vi "Msg.vi"(7 "jettl in":refnum<class "jettl.lvclass">, 11 "Template Msg Strategy in":refnum<class "Template Msg Strategy.lvclass">) -> (5 "jettl out":refnum<class "jettl.lvclass">)   [LabVIEW 2021, in "jettl Msg Template.lvlib" / "Template Msg Strategy.lvclass"]
uses:
  Template Msg Strategy.lvclass
  <vilib>/Nathan Davis/jettl/jettl/jettl/jettl.lvclass
  jettl Msg Template/jettl Msg Template.lvclass
  Template Msg Strategy.lvclass/Template Msg Strategy.ctl
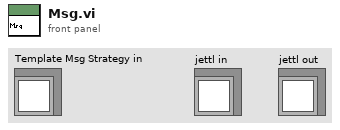
[diagram p1: front panel]
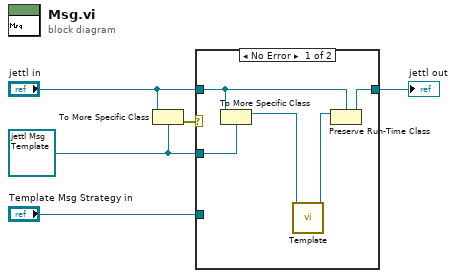
[diagram p0: block diagram]
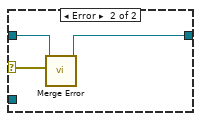
[diagram p2: hidden frame]
diagram:
  w2 = refnum<class "jettl Msg Template.lvclass"> refnum ("jettl Msg Template")
  n1 = To More Specific Class(target class=w2, reference="jettl in") -> (error out=w5:errorcluster)  [unwired: 1 in, 1 out]
  n2 = case shown="No Error" w5 {
    selector: w5 -> [_ w12]
    tunnel: [w8 w11] -> w3
    tunnel: "jettl in" -> [w9 w13]
    tunnel: w2 -> [w10 _]
    tunnel: "Template Msg Strategy in" -> [_ _]
    frame No Error {
      n3 = To More Specific Class(target class=w10, reference=w9) -> (specific class reference=w7:refnum<class "jettl Msg Template.lvclass">)  [unwired: 1 in, 1 out]
      n4 = call-dynamic "Template.vi"("jettl Msg Template in"=w7) -> ("jettl Msg Template out"=w6:refnum<class "jettl Msg Template.lvclass">)  [unwired: 10 in]
      n5 = Preserve Run-Time Class(object in=w6, 2:w9) -> (object out=w8:refnum<class "jettl.lvclass">)  [unwired: 1 in, 1 out]
    }
    frame Error {
      n6 = call-dynamic "Merge Error.vi"("Error"=w12, "jettl Msg Merge Error in"=w13) -> ("jettl Msg Merge Error out"=w11:refnum<class "jettl.lvclass">)  [unwired: 9 in]
    }
  }
  "jettl out" <- w3
